vi "Cubic Spline + Sine Fit Result String.vi"(8 "error in (no error)":errorcluster, 9 "Delta Best Fit Parameters":dbl[](array[numeric]), 10 "Fit Output":T1={"best nonlinear fit"=[], "best fit parameters"=[], "R^2"=0.0, "RMSE"=0.0, "error out"={"status"=FALSE, "code"=0, "source"=""}, "Fitting Method"=enum."Least Square", "number of function calls"=0, "number of iterations"=0, "covariance"=[], "Chi 2"=0.0, "DOF"=0, "Fit Convergence Criterion"=enum."Continue", "Fitting Algorithm"=enum."Levenberg-Marquardt", "Weighted Fit"=enum."Unweighted", "Gradient"=0.0, "|Delta Chi 2|"=0.0, "|Delta Chi 2|/Chi 2"=0.0, "Max |Delta a| /|a|"=0.0, "Lambda"=-1.0, "RSS"=0.0, "AIC"=0.0, "BIC"=0.0, "Max number of function calls"=0, "Max number of iterations"=0, "IRF"={"X Array"=[], "Y Array"=[]}, "IRF Normalization Factor"=0.0, "Decay Normalization Factor"=0.0, "Number of offset fits"=0, "Weighted Chi2"=-1.0, "Unweighted Chi2"=-1.0}) -> (0 "error out":errorcluster, 3 "Result String":string)   [LabVIEW 2021, in "Fits.lvlib"]
uses:
  Fits.lvlib
  Non-linear Fit Output v4.ctl
  Nonlinear Fit Method.ctl
  <vilib>/Analysis/Matrix/Datatypes/RealMatrix.ctl
  Convergence Criteria.ctl
  Non-linear Fitting Algorithm.ctl
  IRF(X)PSED/Fit Weights Type v2.ctl
  Graphs/XY Graph/XY Graph Plot Data.ctl
  <vilib>/Analysis/Matrix/NI_Matrix.lvlib
  Graphs/XY Graph/XY Graph Add-Ons.lvlib
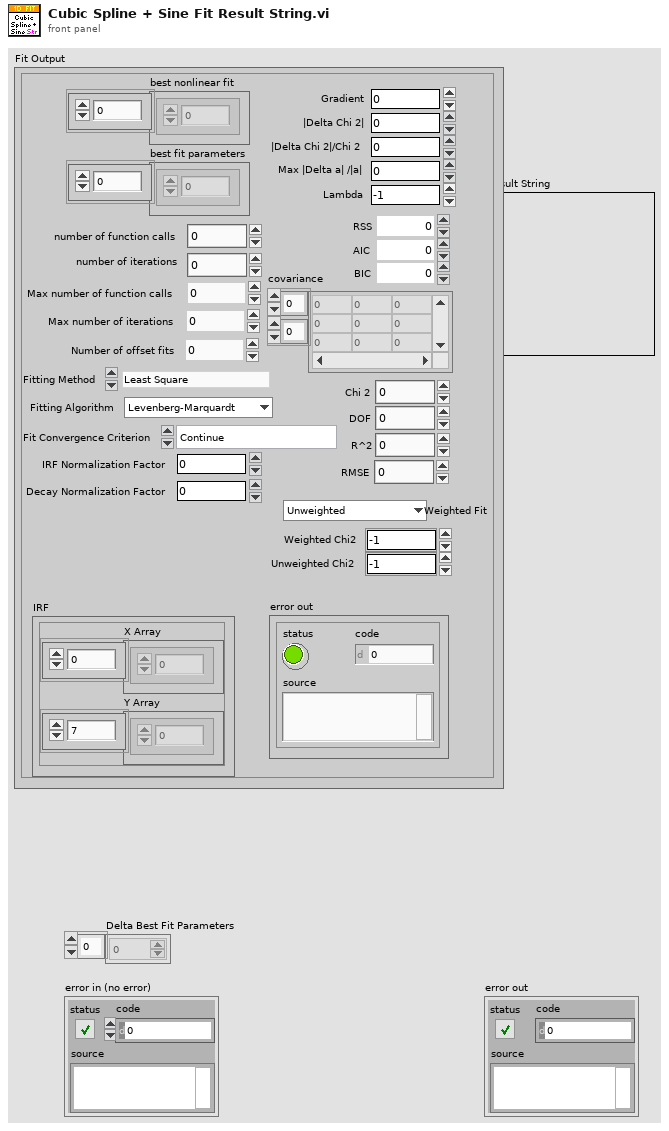
[diagram p1: front panel]
types:
  T1 = typedef "Fits.lvlib/Non-linear Fit Output v4.ctl" = cluster{"best nonlinear fit":dbl[], "best fit parameters":dbl[], "R^2":dbl, "RMSE":dbl, "error out":errorcluster, "Fitting Method":T2, "number of function calls":i32, "number of iterations":i32, "covariance":T3, "Chi 2":dbl, "DOF":i32, "Fit Convergence Criterion":T4, "Fitting Algorithm":T5, "Weighted Fit":T6, "Gradient":dbl, "|Delta Chi 2|":dbl, "|Delta Chi 2|/Chi 2":dbl, "Max |Delta a| /|a|":dbl, "Lambda":dbl, "RSS":dbl, "AIC":dbl, "BIC":dbl, "Max number of function calls":i32, "Max number of iterations":i32, "IRF":T7, "IRF Normalization Factor":dbl, "Decay Normalization Factor":dbl, "Number of offset fits":i32, "Weighted Chi2":dbl, "Unweighted Chi2":dbl}
  T2 = typedef "Fits.lvlib/Nonlinear Fit Method.ctl" = enum16{"Least Square", "Least Absolute Residual", "Bisquare", "MLE"}
  T3 = typedef "NI_Matrix.lvlib/RealMatrix.ctl" = dbl[][]
  T4 = typedef "Fits.lvlib/Convergence Criteria.ctl" = enum16{"Continue", "Tolerances Exceeded", "Max Time Exceeded", "Max Iterations Exceeded", "Max Function Evaluations Exceeded", "Scale Range Exceeded"}
  T5 = typedef "Fits.lvlib/Non-linear Fitting Algorithm.ctl" = enum16{"Levenberg-Marquardt", "Trust-Region Dogleg"}
  T6 = typedef "Fits.lvlib/Fit Weights Type v2.ctl" = enum16{"Unweighted", "1/Variance (Neyman)", "1/Variance (Pearson)", "Best of All"}
  T7 = typedef "XY Graph Add-Ons.lvlib/XY Graph Plot Data.ctl" = cluster{"X Array":dbl[], "Y Array":dbl[]}
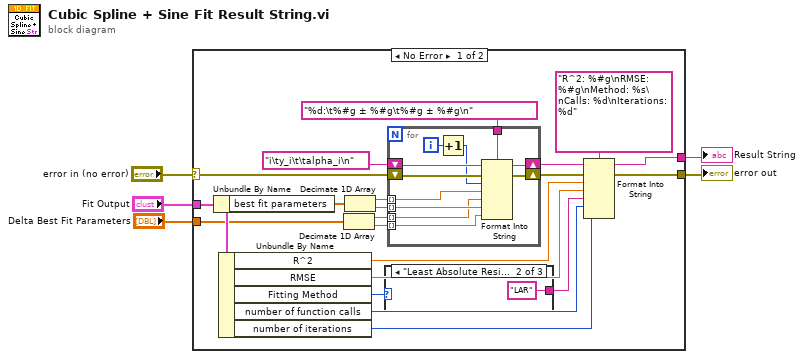
[diagram p0: block diagram]
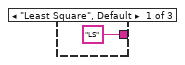
[diagram p2: hidden frame]
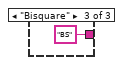
[diagram p3: hidden frame]
diagram:
  n1 = case shown="No Error" "error in (no error)" {
    selector: "error in (no error)" -> [w6 w41]
    tunnel: [w21 w41] -> w4
    tunnel: "Fit Output" -> [w26 _]
    tunnel: "Delta Best Fit Parameters" -> [w7 _]
    tunnel: [w22 _] -> w1
    frame No Error {
      n2 = Unbundle By Name(w26) -> ("best fit parameters"=w8:dbl[])
      n3 = Unbundle By Name(w26) -> ("R^2"=w20:dbl, "RMSE"=w19:dbl, "Fitting Method"=w18:T2, "number of function calls"=w16:i32, "number of iterations"=w15:i32)
      n4 = Decimate 1D Array(w7) -> (w10:dbl[], w9:dbl[])
      n5 = Decimate 1D Array(w8) -> (w14:dbl[], w13:dbl[])
      n6 = case shown="\"Least Absolute Residual\"" w18 {
        tunnel: ["LS" ("input 3") "LAR" ("input 3") "BS" ("input 3")] -> w17
        frame "Least Square", Default {
        }
        frame "Least Absolute Residual" {
        }
        frame "Bisquare" {
        }
      }
      n7 = for {
        tunnel: w14 -> [w36] mode=indexing
        shift-right: [w39] -> w25
        shift-left: "i\ty_i\t\talpha_i\n" ("format string") -> [w40]
        shift-right: [w38] -> w24
        shift-left: w6 -> [w37]
        tunnel: w13 -> [w34] mode=indexing
        tunnel: "%d:\t%#g ± %#g\t%#g ± %#g\n" ("format string") -> [w35]
        tunnel: w10 -> [w33] mode=indexing
        tunnel: w9 -> [w32] mode=indexing
        i -> [w31]
        n8 = Increment(x=w31) -> (x+1=w30:i32)
        n9 = Format Into String(format string=w35, initial string=w40, error in=w37, w30, w36, w33, w34, w32) -> (resulting string=w39:string, error out=w38:errorcluster)
      }
      n10 = Format Into String(format string="R^2: %#g\nRMSE: %#g\nMethod: %s\nCalls: %d\nIterations: %d", initial string=w25, error in=w24, w20, w19, w17, w16, w15) -> (resulting string=w22:string, error out=w21:errorcluster)
    }
    frame Error {
    }
  }
  "Result String" <- w1
  "error out" <- w4
